vi "Backward Decompose Number.VI"(0 "number as string":string) -> (1 "string start":string, 2 "string rest":string)   [LabVIEW 2017, in "NI_Gmath.lvlib"]
uses:
  <vilib>/gmath/NI_Gmath.lvlib
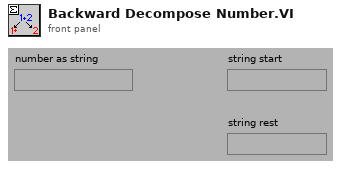
[diagram p1: front panel]
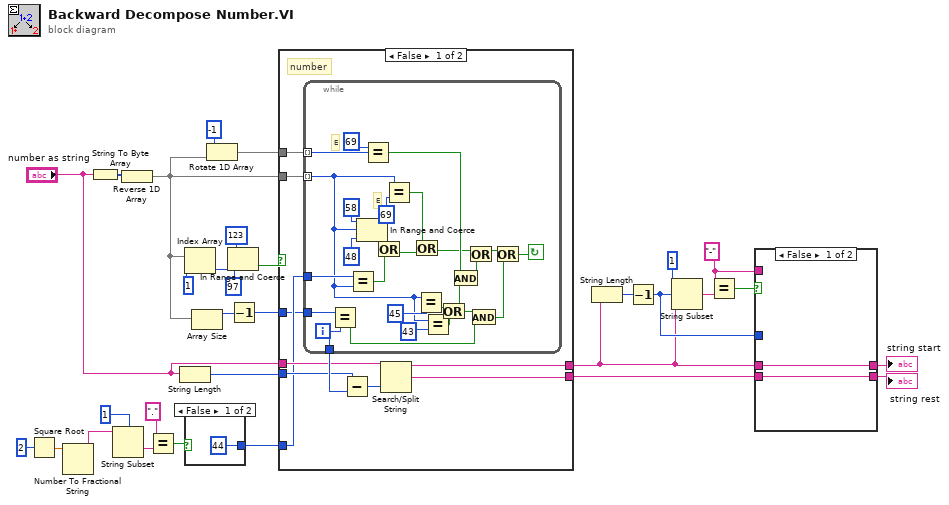
[diagram p0: block diagram]
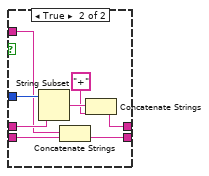
[diagram p2: hidden frame]
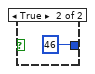
[diagram p3: hidden frame]
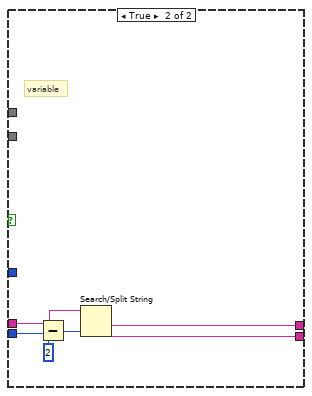
[diagram p4: hidden frame]
diagram:
  w1 = "-"
  w26 = 1
  n1 = Square Root(x=2) -> (sqrt(x)=w24:dbl)
  n2 = Number To Fractional String(number=w24) -> (F-format string=w27:string)  [unwired: 3 in]
  n3 = String To Byte Array(string="number as string") -> (unsigned byte array=w31:u8[])
  n4 = String Subset(string=w27, offset (0)=w26, length (rest)=w26) -> (substring=w23:string)
  n5 = Reverse 1D Array(array=w31) -> (reversed array=w13:u8[])
  n6 = Equal?(x=".", y=w23) -> (x = y?=w21:bool)
  n7 = String Length(string="number as string") -> (length=w29:i32)
  n8 = Index Array(array=w13, index=1) -> (element=w19:u8)
  n9 = case shown="False" w21 {
    tunnel: [44 46] -> w20
    frame False {
    }
    frame True {
    }
  }
  n10 = Array Size(array=w13) -> (size(s)=w12:i32)
  n11 = Rotate 1D Array(1:w13, 2:-1) -> (0:w14:u8[])
  n12 = In Range and Coerce(upper limit=123, x=w19, lower limit=97) -> (In Range?=w16:bool)  [unwired: 1 out]
  n13 = Decrement(x=w12) -> (x-1=w11:i32)
  n14 = case shown="False" w16 {
    tunnel: w29 -> [w42 w74]
    tunnel: "number as string" -> [w41 w69]
    tunnel: [w39 w71] -> w3
    tunnel: [w38 w70] -> w5
    tunnel: w20 -> [w37 _]
    tunnel: w13 -> [w36 _]
    tunnel: w14 -> [w35 _]
    tunnel: w11 -> [w34 _]
    frame False {
      # "number"
      n15 = while {
        tunnel: w34 -> [w46]
        tunnel: w35 -> [w57] mode=indexing
        tunnel: w36 -> [w55] mode=indexing
        tunnel: w37 -> [w65]
        tunnel: [w66] -> w43
        i -> [w66]
        stop <- w47 continue-if-true
        # "E"
        # "E"
        n16 = Equal?(x=w46, y=w66) -> (x = y?=w45:bool)
        n17 = Equal?(x=w65, y=w55) -> (x = y?=w67:bool)
        n18 = In Range and Coerce(upper limit=58, x=w55, lower limit=48) -> (In Range?=w68:bool)  [unwired: 1 out]
        n19 = Equal?(x=69, y=w57) -> (x = y?=w56:bool)
        n20 = Or(x=w68, y=w67) -> (x .or. y?=w53:bool)
        n21 = Equal?(x=w55, y=69) -> (x = y?=w52:bool)
        n22 = Or(x=w52, y=w53) -> (x .or. y?=w51:bool)
        n23 = Equal?(x=w55, y=45) -> (x = y?=w61:bool)
        n24 = Equal?(x=w55, y=43) -> (x = y?=w62:bool)
        n25 = Or(x=w61, y=w62) -> (x .or. y?=w50:bool)
        n26 = And(x=w56, y=w50) -> (x .and. y?=w49:bool)
        n27 = Or(x=w51, y=w49) -> (x .or. y?=w48:bool)
        n28 = And(x=w50, y=w45) -> (x .and. y?=w44:bool)
        n29 = Or(x=w48, y=w44) -> (x .or. y?=w47:bool)
      }
      n30 = Subtract(x=w42, y=w43) -> (x-y=w40:i32)
      n31 = Search/Split String(string=w41, offset (0)=w40) -> (substring before match=w39:string, match + rest of string=w38:string)  [unwired: 1 in, 1 out]
    }
    frame True {
      # "variable"
      n32 = Subtract(x=w74, y=2) -> (x-y=w72:i32)
      n33 = Search/Split String(string=w69, offset (0)=w72) -> (substring before match=w71:string, match + rest of string=w70:string)  [unwired: 1 in, 1 out]
    }
  }
  n34 = String Length(string=w3) -> (length=w10:i32)
  n35 = Decrement(x=w10) -> (x-1=w9:i32)
  n36 = String Subset(string=w3, offset (0)=w9, length (rest)=1) -> (substring=w7:string)
  n37 = Equal?(x=w1, y=w7) -> (x = y?=w6:bool)
  n38 = case shown="False" w6 {
    tunnel: w5 -> [w76 w81]
    tunnel: [w76 w84] -> w4
    tunnel: w3 -> [w75 w82]
    tunnel: [w75 w77] -> w2
    tunnel: w1 -> [_ w80]
    tunnel: w9 -> [_ w83]
    frame False {
    }
    frame True {
      n39 = String Subset(string=w82, length (rest)=w83) -> (substring=w79:string)  [unwired: 1 in]
      n40 = Concatenate Strings(w80, w81) -> (w84:string)
      n41 = Concatenate Strings(w79, "+") -> (w77:string)
    }
  }
  "string start" <- w2
  "string rest" <- w4
